vi "Kalman_smoothing_V1.vi"() -> ()   [LabVIEW 2019]
panel:
  out "Filtered":dbl(slide) scale=-20.0..20.0
  out "Compare":cluster{dbl, "data":dbl}(graph)
  in  "weighting term":dbl
  out "Raw Data":dbl(slide) scale=-20.0..20.0
  in  "stop 2":bool
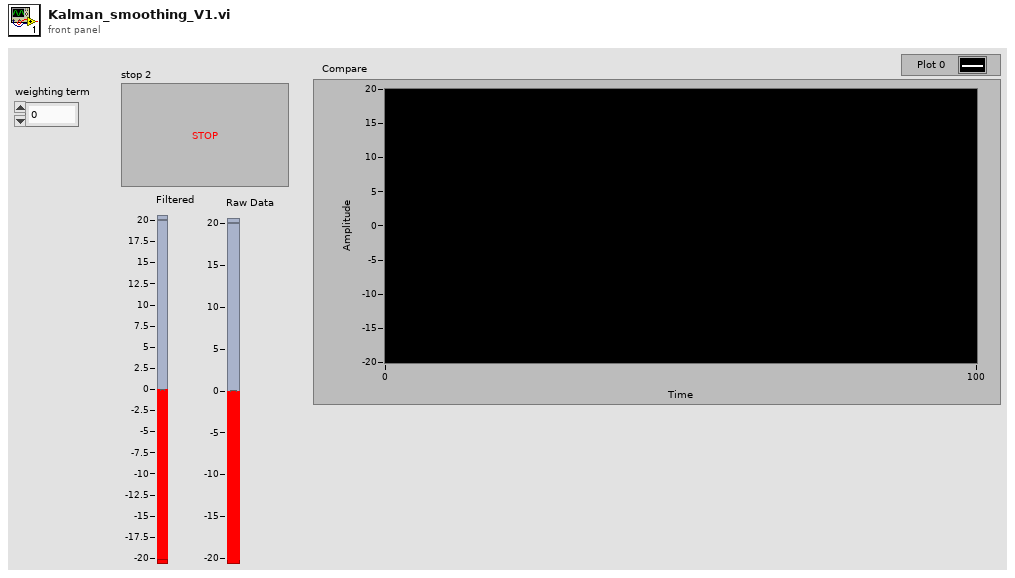
[diagram p1: front panel]
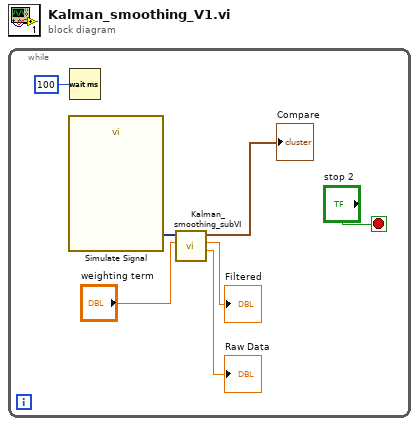
[diagram p0: block diagram]
diagram:
  n1 = while {
    stop <- "stop 2" stop-if-true
    n2 = call "Simulate Signal"() -> ("Sine with Uniform Noise"=w6:dynamicdata)  [unwired: 14 in, 1 out]
    n3 = Wait (ms)(milliseconds to wait=u32 100) -> ()  [unwired: 1 out]
    n4 = call "Kalman_smoothing_subVI.vi"("weighting term"="weighting term", "Signal with  Noise"=w6) -> ("Raw Data"=→"Raw Data":dbl, "Filtered"=→"Filtered":dbl, "Compare"=→"Compare":cluster{dbl, "data":dbl})  [unwired: 7 in]
  }
